vi "_Josep_curr_Imag_2.vi"(9 "Joseph_curr":T2={"start(mA)"=0.0, "stop(mA)"=20.0, "step(mA)"=1.0, "file_name"="JC_874.00_121_110803_deflux_P1.csv", "パス"=path "C:/Documents and Settings/band10/デスクトップ/data/cartridge/CCA02/CCA02-02/Deflux", "save?"=TRUE, "SIS Bias range Vsis"={"start"=-0.1, "stop"=0.1, "step"=0.02}}, 11 "Bias_LO_equip":T1={"Node address"=19, "CAN Interface"="CAN0", "Cartridge band"=10, "Slave Node in"={"Address"=19, "Serial Number"=[16, -88, -112, 75, 1, 8, 0, 24]}, "ObjHandle out"=93192256, "POL"=1, "sb"=1, "GPIB_SM (SIS S,V)"="24", "GPIB_DMM (SIS I)"="22", "GPIB_SM (MAG I) "="25", "GPIB_SG(LO)"="19", "GPIB_PW (PAMP) "="6", "GPIB_TMP1(8ch)"="12", "GPIB_TMP2(2ch)  "="13", "WCA_avg"=10, "Rsen"=10.0, "BiasModule"=1, "LOModule "=2, "WCA_LO_FREQ_SET"={"YTO Low freq. [GHz]"=14.66, "YTO High freq. [GHz]"=17.5, "Kvco"=1, "Lock Pol."=0, "SET LO FREQ"=97.111115, "Multiplier"=6.0, "YTO (HEX)"=2189, "YTO coarse( FREQ)"=16.178135, "NULL PLL INTEGRATOR"=FALSE}, "Res for"=0} {"Res for" items=["none", "series res", "parallel res"]; "WCA_LO_FREQ_SET"."YTO coarse( FREQ)" min=25 max=150 step=0.0001 format="%.3f"; "WCA_LO_FREQ_SET"."Multiplier" min=3 max=6 step=3; "WCA_LO_FREQ_SET"."SET LO FREQ" min=25 max=150 step=0.0001 format="%.3f"; "WCA_LO_FREQ_SET"."Lock Pol." items=["Lower", "Upper"]; "WCA_LO_FREQ_SET"."Kvco" items=["7.5MHz/V", "15MHz/V"]; "WCA_LO_FREQ_SET"."YTO High freq. [GHz]" format="%.3f"; "WCA_LO_FREQ_SET"."YTO Low freq. [GHz]" format="%.3f"; "LOModule" items=["Manual", "B10Lab LO", "WCA LO"]; "BiasModule" items=["B10Lab Bias", "WCA BiasModule"]; "Slave Node in"."Serial Number" format="%.0x"; "Slave Node in"."Address" format="%.0x"; "Cartridge band" max=10 step=1; "Node address" format="%.0x"}) -> ()   [LabVIEW 2017]
uses:
  __sub_vi/WCA_NAOJ_sub_vi/WCA_Global.vi
  <vilib>/express/express arith-compare/Formula/XNode/ExpressFormulaBlockNode.xnode
panel:
  in  "time1":i32=1000
  in  "Time0":i32=1000
  in  "set0?":bool=TRUE
  out "Link済み 2":bool=TRUE
  out "Link済み":bool=TRUE
  out "XYグラフ 2":cluster{dbl[], dbl[]}(graph)={[0.0, 1.0, 2.0, 3.0, 4.0, 5.0, 6.0, 7.0, 8.0, 9.0, 10.0, 11.0, 12.0, 13.0, 14.0, 15.0, 16.0, 17.0, 18.0, 19.0, 20.0], [47.265625, 48.779296875, 45.635986328125, 36.9659423828125, 23.81591796875, 11.5509033203125, 2.508544921875, 11.7523193359375, 12.109375, 6.5277099609375, 1.5167236328125, 3.3172607421875, 4.6142578125, 3.216552734375, 1.5106201171875, 2.3406982421875, 2.8564453125, 2.52685546875, 2.1514892578125, 1.458740234375, 1.5594482421875]}
  # "LO freq. [GHz]"
  # "YTO LOW\n/High Freq."
  # "ZERO Intgrtr"
  # "Node Address"
  # "Serial Number"
  # "Magnet current"
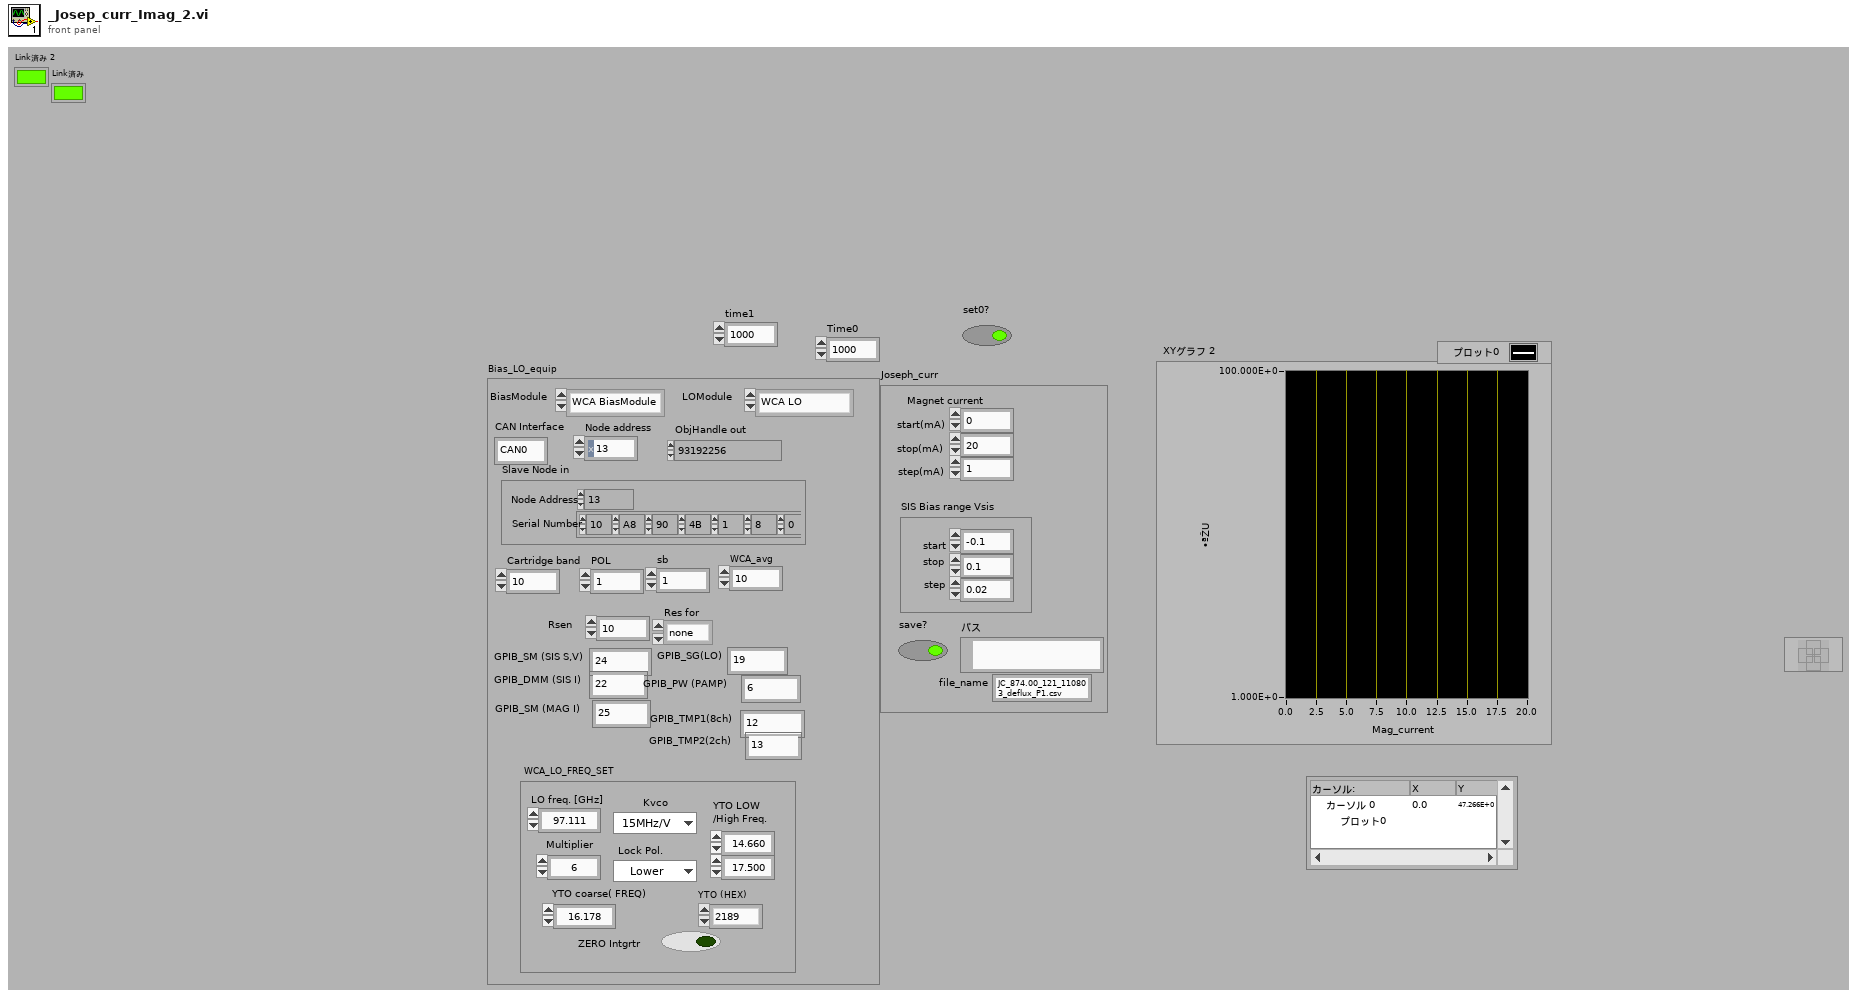
[diagram p1: front panel]
types:
  T1 = cluster{"Node address":u16, "CAN Interface":string, "Cartridge band":u32, "Slave Node in":cluster{"Address":i16, "Serial Number":i8[]}, "ObjHandle out":u32, "POL":u32, "sb":u32, "GPIB_SM (SIS S,V)":string, "GPIB_DMM (SIS I)":string, "GPIB_SM (MAG I) ":string, "GPIB_SG(LO)":string, "GPIB_PW (PAMP) ":string, "GPIB_TMP1(8ch)":string, "GPIB_TMP2(2ch)  ":string, "WCA_avg":i32, "Rsen":dbl, "BiasModule":u16, "LOModule ":u16, "WCA_LO_FREQ_SET":cluster{"YTO Low freq. [GHz]":sgl, "YTO High freq. [GHz]":sgl, "Kvco":u16, "Lock Pol.":u16, "SET LO FREQ":sgl, "Multiplier":sgl, "YTO (HEX)":u16, "YTO coarse( FREQ)":sgl, "NULL PLL INTEGRATOR":bool}, "Res for":u16}
  T2 = cluster{"start(mA)":dbl, "stop(mA)":dbl, "step(mA)":dbl, "file_name":string, "パス":path, "save?":bool, "SIS Bias range Vsis":cluster{"start":dbl, "stop":dbl, "step":dbl}}
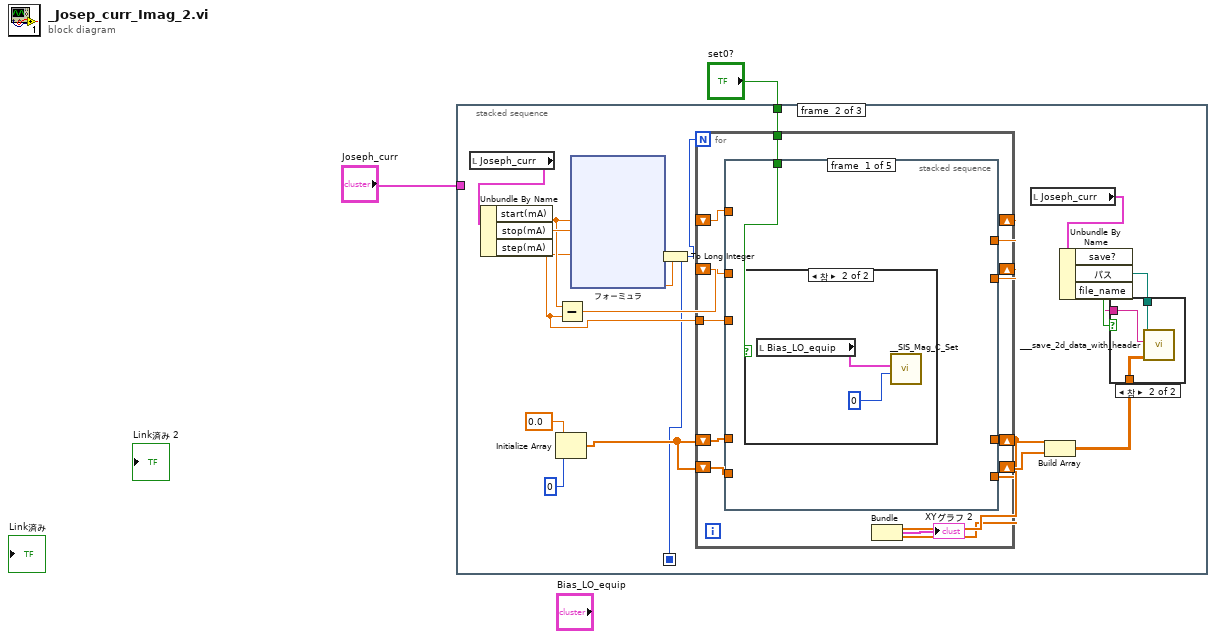
[diagram p0: block diagram]
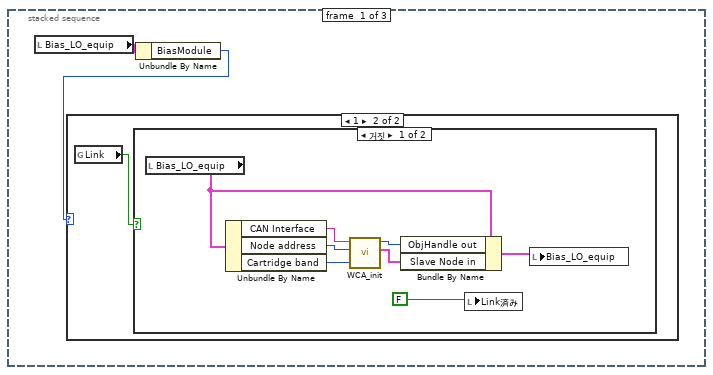
[diagram p2: hidden frame]
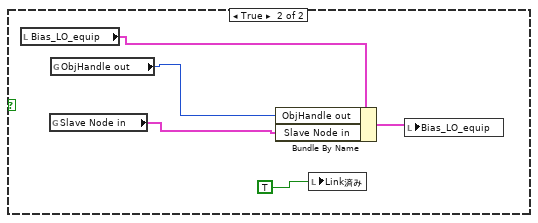
[diagram p4: hidden frame]
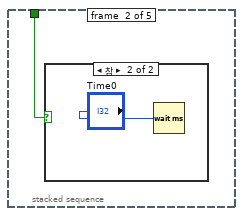
[diagram p7: hidden frame]
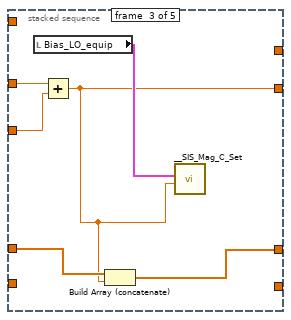
[diagram p9: hidden frame]
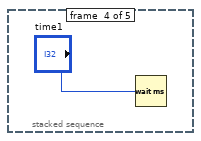
[diagram p10: hidden frame]
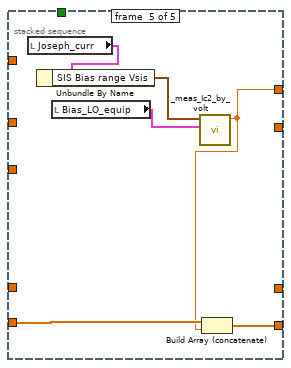
[diagram p11: hidden frame]
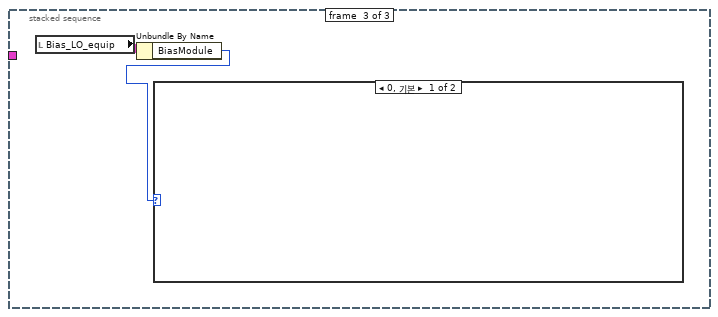
[diagram p12: hidden frame]
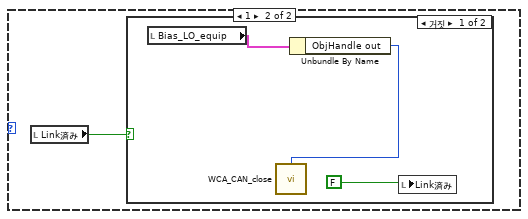
[diagram p13: hidden frame]
diagram:
  n1 = stacked-sequence {
    seq-local: [_ w25 _] -> [_ _ _]
    tunnel: "Joseph_curr" -> [_ _ _]
    tunnel: "set0?" -> [_ w21 _]
    frame #0 {
      n2 = local read "Bias_LO_equip"() -> (w4:T1)
      n3 = Unbundle By Name(w4) -> ("BiasModule"=w3:u16)
      n4 = case shown="1" w3 {
        frame 0, Default {
        }
        frame 1 {
          n5 = global read "WCA_Global.vi" "Link"() -> (w5:bool)
          n6 = case shown="거짓" w5 {
            frame False {
              n7 = local read "Bias_LO_equip"() -> (w6:T1)
              n8 = Unbundle By Name(w6) -> ("CAN Interface"=w10:string, "Node address"=w9:u16, "Cartridge band"=w8:u32)
              n9 = call "WCA_init.vi"("Cartridge band"=w8, "Node address"=w9, "CAN Interface"=w10) -> ("Slave Node in"=w12:cluster{"Address":i16, "Serial Number":i8[]}, "ObjHandle out"=w13:u32)  [unwired: 4 in, 3 out]
              n10 = Bundle By Name(cluster=w6, "ObjHandle out"=w13, "Slave Node in"=w12) -> (w7:T1)
              n11 = local write "Link済み"(FALSE) -> ()
              n12 = local write "Bias_LO_equip"(w7) -> ()
            }
            frame True {
              n13 = local read "Bias_LO_equip"() -> (w17:T1)
              n14 = global read "WCA_Global.vi" "Slave Node in"() -> (w15:cluster{"Address":i16, "Serial Number":i8[]})
              n15 = global read "WCA_Global.vi" "ObjHandle out"() -> (w16:u32)
              n16 = Bundle By Name(cluster=w17, "ObjHandle out"=w16, "Slave Node in"=w15) -> (w18:T1)
              n17 = local write "Link済み"(TRUE) -> ()
              n18 = local write "Bias_LO_equip"(w18) -> ()
            }
          }
        }
      }
    }
    frame #1 {
      n19 = local read "Joseph_curr"() -> (w36:T2)
      n20 = Unbundle By Name(w36) -> ("start(mA)"=w33:dbl, "stop(mA)"=w35:dbl, "step(mA)"=w31:dbl)
      n21 = Initialize Array(0.0, 0) -> (w28:dbl[])
      n22 = Subtract(x=w33, y=w31) -> (x-y=w32:dbl)
      n23 = xnode "フォーミュラ"("start"=w33, "stop"=w35, "step"=w31) -> ("結果"=w34:dbl)  [unwired: 1 in, 1 out]
      n24 = To Long Integer(number=w34) -> (32bit integer=w25:i32)
      n25 = for {
        N: w25 -> [_]
        shift-right: [w60] -> _
        shift-left: w32 -> [w62]
        tunnel: w31 -> [w61]
        shift-right: [w56] -> w27
        shift-left: w28 -> [w59]
        shift-right: [w55] -> w26
        shift-left: w28 -> [w58]
        shift-right: [w53] -> _
        shift-left: _ -> [w54]
        tunnel: w21 -> [w52]
        n26 = stacked-sequence {
          tunnel: w62 -> [_ _ w73 _ _]
          tunnel: w61 -> [_ _ w72 _ _]
          tunnel: [_ _ w68 _ _] -> w60
          tunnel: w59 -> [_ _ w71 _ _]
          tunnel: [_ _ w70 _ _] -> w56
          tunnel: w58 -> [_ _ _ _ w80]
          tunnel: [_ _ _ _ w79] -> w55
          tunnel: w54 -> [_ _ _ _ _]
          tunnel: [_ _ _ _ w78] -> w53
          tunnel: w52 -> [w63 w66 _ _ _]
          frame #0 {
            n27 = case shown="참" w63 {
              frame False {
              }
              frame True {
                n28 = local read "Bias_LO_equip"() -> (w65:T1)
                n29 = call "__SIS_Mag_C_Set.vi"("Set_Mag_C"=0, "Bias_LO_equip"=w65) -> ()  [unwired: 10 in]
              }
            }
          }
          frame #1 {
            n30 = case shown="참" w66 {
              frame False {
              }
              frame True {
                n31 = Wait (ms)(milliseconds to wait="Time0") -> ()  [unwired: 1 out]
              }
            }
          }
          frame #2 {
            n32 = local read "Bias_LO_equip"() -> (w69:T1)
            n33 = Add(x=w73, y=w72) -> (x+y=w68:dbl)
            n34 = Build Array (concatenate)(w71, w68) -> (w70:dbl[])
            n35 = call "__SIS_Mag_C_Set.vi"("Set_Mag_C"=w68, "Bias_LO_equip"=w69) -> ()  [unwired: 10 in]
          }
          frame #3 {
            n36 = Wait (ms)(milliseconds to wait="time1") -> ()  [unwired: 1 out]
          }
          frame #4 {
            n37 = local read "Joseph_curr"() -> (w76:T2)
            n38 = Unbundle By Name(w76) -> ("SIS Bias range Vsis"=w75:cluster{"start":dbl, "stop":dbl, "step":dbl})
            n39 = local read "Bias_LO_equip"() -> (w77:T1)
            n40 = call "_meas_Ic2_by_volt.vi"("Bias_LO_equip"=w77, "Icクラスタ"=w75) -> ("IC"=w78:dbl)  [unwired: 5 in]
            n41 = Build Array (concatenate)(w80, w78) -> (w79:dbl[])
          }
        }
        n42 = Bundle(w56, w55) -> (→"XYグラフ 2":cluster{dbl[], dbl[]})  [unwired: 1 in]
      }
      n43 = local read "Joseph_curr"() -> (w23:T2)
      n44 = Build Array(w27, w26) -> (w24:dbl[][])
      n45 = Unbundle By Name(w23) -> ("save?"=w22:bool, "パス"=w20:path, "file_name"=w19:string)
      n46 = case shown="참" w22 {
        tunnel: w24 -> [_ w51]
        tunnel: w20 -> [_ w50]
        tunnel: w19 -> [_ w49]
        frame False {
        }
        frame True {
          n47 = call "___save_2d_data_with_header.vi"("配列"=w51, "file_name"=w49, "パス"=w50) -> ()  [unwired: 8 in, 1 out]
        }
      }
    }
    frame #2 {
      n48 = local read "Bias_LO_equip"() -> (w82:T1)
      n49 = Unbundle By Name(w82) -> ("BiasModule"=w81:u16)
      n50 = case shown="0, 기본" w81 {
        frame 0, Default {
        }
        frame 1 {
          n51 = local read "Link済み"() -> (w83:bool)
          n52 = case shown="거짓" w83 {
            frame False {
              n53 = local read "Bias_LO_equip"() -> (w85:T1)
              n54 = Unbundle By Name(w85) -> ("ObjHandle out"=w84:u32)
              n55 = call "WCA_CAN_close.vi"("ObjHandle in"=w84) -> ()  [unwired: 14 in, 1 out]
              n56 = local write "Link済み"(FALSE) -> ()
            }
            frame True {
            }
          }
        }
      }
    }
  }
